vi "OSIPI OPCUA Server.vi"(11 "Main Queue Cluster":T1) -> ()   [LabVIEW 2018]
uses:
  <vilib>/OPCUA/controls/Supported Security Policies.ctl
  Drag and Drop/State Cluster.ctl
  support/Message Queue/Message Cluster.ctl
  Drag and Drop/Thumbnail Cluster.ctl
  Drag and Drop/Object Cluster.ctl
  <vilib>/Utility/miscctls.llb/LVRectTypeDef.ctl
  Drag and Drop/Object Type Enum.ctl
  <vilib>/Utility/miscctls.llb/LVPositionTypeDef.ctl
  Config Module/Controls/Main Config Cluster.ctl
  OPC Module Config.ctl
  Scale Module Folder/Measure Instrument/State Enum.ctl
  <vilib>/Utility/miscctls.llb/LVPoint32TypeDef.ctl
  OPC Settings.ctl
  Variable Data Cluster.ctl
  <vilib>/OPCUA/controls/NodeId.ctl
  <vilib>/OPCUA/controls/OPC UA StatusCode.ctl
  <vilib>/OPCUA/controls/Subscription ID.ctl
  <vilib>/OPCUA/controls/OPC UA Client Refnum.ctl
  <vilib>/OPCUA/controls/Subscription Data Change.ctl
  <vilib>/OPCUA/controls/Data Type.ctl
  Feed Module/Controls/Feed Module Config Cluster.ctl
  Feed Module/Controls/Feed Module Settings Cluster.ctl
  Ismatec ISM 831C/Controls/Ismatech Settings Cluster.ctl
  Masterflex 7550-30/Controls/Settings Cluster.ctl
  Mettler Toledo/Controls/Settings Cluster.ctl
  Bronkhorst M13 Flow Meter/Settings Cluster.ctl
  Measure Instrument/PID 2 Parameters Cluster.ctl
  Measure Instrument/PID Input Enum.ctl
  Measure Instrument/PID 2 Output Enum.ctl
  Tacmina QI/Tacmina QI DAQ Setting.ctl
  KNF Pump/Settings Cluster plus SIMDOS.ctl
  ASIA Pump/Pump Settings.ctl
  VICI M50 Party Mode/Settings Cluster.ctl
  FLOM Pump/Settings Cluster.ctl
  SSI PR Class/SSI PR or LD Settings Cluster.ctl
  Masterflex 75211/Masterflex 75211 DAQ Setting.ctl
  SSI PR Class/SSI P40 Settings Cluster.ctl
  TT Module/Controls/TT Module Config Cluster.ctl
  Tag VIs/Numeric Alarm Settings Cluster.ctl
  Acquisition/Hardware Configuration.ctl
  Acquisition/Task Cluster.ctl
  PT Module/Controls/PT Module Config Cluster.ctl
  Scale Module Folder/Feed Module/Controls/Scale Module Config Cluster.ctl
  Scale Module Folder/Feed Module/Controls/Scale Module Settings Cluster.ctl
  Pump Module Folder/Pump Module Config Cluster.ctl
  Pump Module Folder/Pump Module Settings Cluster.ctl
  LabJack Module/Controls/U3 Module Config Cluster.ctl
  Decoration Module/Decoration Module Config Cluster.ctl
  Flow Module Folder/Feed Module/Controls/Flow Module Config Cluster.ctl
  Flow Module Folder/Feed Module/Controls/Flow Module Settings Cluster.ctl
  TCU Module/TCU Module Folder/TCU Module Config Cluster.ctl
  TCU Module/TCU Module Folder/TCU Module Settings Cluster.ctl
  TCU Module/TCU Module Folder/Measure Instrument/Output Devices.ctl
  Huber TCU/Huber Settings.ctl
  Lauda Integral XT-150 TCU/Lauda Settings.ctl
  Julabo Type 1 TCU/Julabo Type 1 TCU Folder/Julabo FP-50 Settings.ctl
  Huber Unistat 410 TCU/Huber Unistat 410 RS485 Settings.ctl
  D-O Module Folder/Not Sure Where this is Used.ctl
  Sequencing/Squence Control.ctl
  D-O Module Folder/D-O Module Config Cluster.ctl
  D-O Module Folder/Valve Clusters.ctl
  D-O Module Folder/D-O Module Settings Cluster.ctl
  D-O Module Folder/D-O Device Settings Cluster.ctl
  VICI Electronic Actuator/VICI Electronic Actuator Settings.ctl
  Pressure Regulator Control Module/Pressure Regulator/Controls/4-20mA Module Config Cluster.ctl
  Pressure Regulator Control Module/Pressure Regulator/Controls/4-20mA Module Settings Cluster.ctl
  Pressure Transmitter/Pressure Transmitter Device Settings.ctl
  Pressure Reg Module/Pressure Regulator Device Settings.ctl
  <vilib>/OPCUA/controls/OPC UA Variable Node Refnum.ctl
  <vilib>/OPCUA/controls/OPC UA Server Refnum.ctl
  Main/Main Queue Cluster.ctl
  Tag VIs/Tag FGV Operation Enum.ctl
  <vilib>/OPCUA/server/Write Double.vi
  <vilib>/OPCUA/NI OPC UA Server.lvlib
  support/Message Queue/Message Queue.lvlib
  Shared Variables/Dynamic Shared Variables.lvlib
  support/Message Queue/Enqueue Message (Single).vi
  TT Module/TT Module.lvlib
  Masterflex 7550-30/Masterflex 7550-30.lvlib
  Ismatec ISM 831C/Ismatec ISM 831C.lvlib
  Tacmina QI/Tacmina QI.lvlib
  KNF Pump/KNF SIMDOS.lvlib
  VICI M50 Party Mode/VICI M6 M50 Party Mode.lvlib
  FLOM Pump/FLOM Pump.lvlib
  ASIA Pump.lvlib
  Mettler Toledo/Mettler Toledo.lvlib
  Bronkhorst M13 Flow Meter/Bronkhorst M13 Flow Meter.lvlib
  SSI PR Class/SSI PR or LD Pump.lvlib
  Feed Module/Feed Module.lvlib
  DAQ/DAQ.lvlib
  PT Module/PT Module.lvlib
  Scale Module Folder/Scale Module.lvlib
  Pump Module Folder/Pump Module.lvlib
  LabJack Module/U3 Module.lvlib
  Flow Module Folder/Flow Module.lvlib
  Huber TCU/Huber Ministat 230 TCU.lvlib
  Lauda Integral XT-150 TCU/Lauda TCU.lvlib
  Julabo Type 1 TCU/Julabo Type 1 TCU Folder/Julabo Type FP-50 TCU.lvlib
  TCU Module/TCU Module Folder/TCU Module.lvlib
  Sequencing/Sequencing Library.lvlib
  D-O Module Folder/D-O Module.lvlib
  Pressure Transmitter/Pressure Transmitter Library.lvlib
  Pressure Reg Module/Pressure Regulator Library.lvlib
  Pressure Regulator Control Module/Pressure Regulator/4-20mA Module.lvlib
  OPC UA.lvlib
  Scale Module Folder/Measure Instrument/Scale Module Engine.lvlib
  Config Module/Config Module.lvlib
  Drag and Drop/Drag and Drop.lvlib
  D-O Module Folder/DIO Valve/VICI Electronic Actuator.lvlib
  Masterflex 75211/Masterflex 75211.lvlib
  SSI PR Class/SSI P40 Pump.lvlib
  Huber Unistat 410 TCU/Huber Unistat 410 TCU.lvlib
panel:
  out "Array 3":T4(array[cluster])
  out "OPC UA server refnum out 3":T5
  out "Array 2":T6[](array[typedef]) items=["Good"=0, "Good_SubscriptionTransferred"=2949120, "Good_CompletesAsynchronously"=3014656, "Good_Overload"=3080192, "Good_Clamped"=3145728, "Good_LocalOverride"=9830400, "Good_EntryInserted"=10616832, "Good_EntryReplaced"=10682368, "Good_NoData"=10813440, "Good_MoreData"=10878976, "Good_CommunicationEvent"=10944512, "Good_ShutdownEvent"=11010048, "Good_CallAgain"=11075584, "Good_NonCriticalTimeout"=11141120, "Good_ResultsMayBeIncomplete"=12189696, "Good_DataIgnored"=14221312, "Uncertain"=1073741824, "Uncertain_ReferenceOutOfServer"=1080819712, "Uncertain_NoCommunicationLastUsableValue"=1083113472, "Uncertain_LastUsableValue"=1083179008, "Uncertain_SubstituteValue"=1083244544, "Uncertain_InitialValue"=1083310080, "Uncertain_SensorNotAccurate"=1083375616, "Uncertain_EngineeringUnitsExceeded"=1083441152, "Uncertain_SubNormal"=1083506688, "Uncertain_DataSubNormal"=1084489728, "Uncertain_ReferenceNotDeleted"=1086062592, "Uncertain_NotAllNodesAvailable"=1086324736, "Bad"=2147483648, "Bad_UnexpectedError"=2147549184, "Bad_InternalError"=2147614720, "Bad_OutOfMemory"=2147680256, "Bad_ResourceUnavailable"=2147745792, "Bad_CommunicationError"=2147811328, "Bad_EncodingError"=2147876864, "Bad_DecodingError"=2147942400, "Bad_EncodingLimitsExceeded"=2148007936, "Bad_UnknownResponse"=2148073472, "Bad_Timeout"=2148139008, "Bad_ServiceUnsupported"=2148204544, "Bad_Shutdown"=2148270080, "Bad_ServerNotConnected"=2148335616, "Bad_ServerHalted"=2148401152, "Bad_NothingToDo"=2148466688, "Bad_TooManyOperations"=2148532224, "Bad_DataTypeIdUnknown"=2148597760, "Bad_CertificateInvalid"=2148663296, "Bad_SecurityChecksFailed"=2148728832, "Bad_CertificateTimeInvalid"=2148794368, "Bad_CertificateIssuerTimeInvalid"=2148859904, "Bad_CertificateHostNameInvalid"=2148925440, "Bad_CertificateUriInvalid"=2148990976, "Bad_CertificateUseNotAllowed"=2149056512, "Bad_CertificateIssuerUseNotAllowed"=2149122048, "Bad_CertificateUntrusted"=2149187584, "Bad_CertificateRevocationUnknown"=2149253120, "Bad_CertificateIssuerRevocationUnknown"=2149318656, "Bad_CertificateRevoked"=2149384192, "Bad_CertificateIssuerRevoked"=2149449728, "Bad_UserAccessDenied"=2149515264, "Bad_IdentityTokenInvalid"=2149580800, "Bad_IdentityTokenRejected"=2149646336, "Bad_SecureChannelIdInvalid"=2149711872, "Bad_InvalidTimestamp"=2149777408, "Bad_NonceInvalid"=2149842944, "Bad_SessionIdInvalid"=2149908480, "Bad_SessionClosed"=2149974016, "Bad_SessionNotActivated"=2150039552, "Bad_SubscriptionIdInvalid"=2150105088, "Bad_RequestHeaderInvalid"=2150236160, "Bad_TimestampsToReturnInvalid"=2150301696, "Bad_RequestCancelledByClient"=2150367232, "Bad_NoCommunication"=2150694912, "Bad_WaitingForInitialData"=2150760448, "Bad_NodeIdInvalid"=2150825984, "Bad_NodeIdUnknown"=2150891520, "Bad_AttributeIdInvalid"=2150957056, "Bad_IndexRangeInvalid"=2151022592, "Bad_IndexRangeNoData"=2151088128, "Bad_DataEncodingInvalid"=2151153664, "Bad_DataEncodingUnsupported"=2151219200, "Bad_NotReadable"=2151284736, "Bad_NotWritable"=2151350272, "Bad_OutOfRange"=2151415808, "Bad_NotSupported"=2151481344, "Bad_NotFound"=2151546880, "Bad_ObjectDeleted"=2151612416, "Bad_NotImplemented"=2151677952, "Bad_MonitoringModeInvalid"=2151743488, "Bad_MonitoredItemIdInvalid"=2151809024, "Bad_MonitoredItemFilterInvalid"=2151874560, "Bad_MonitoredItemFilterUnsupported"=2151940096, "Bad_FilterNotAllowed"=2152005632, "Bad_StructureMissing"=2152071168, "Bad_EventFilterInvalid"=2152136704, "Bad_ContentFilterInvalid"=2152202240, "Bad_FilterOperandInvalid"=2152267776, "Bad_ContinuationPointInvalid"=2152333312, "Bad_NoContinuationPoints"=2152398848, "Bad_ReferenceTypeIdInvalid"=2152464384, "Bad_BrowseDirectionInvalid"=2152529920, "Bad_NodeNotInView"=2152595456, "Bad_ServerUriInvalid"=2152660992, "Bad_ServerNameMissing"=2152726528, "Bad_DiscoveryUrlMissing"=2152792064, "Bad_SempahoreFileMissing"=2152857600, "Bad_RequestTypeInvalid"=2152923136, "Bad_SecurityModeRejected"=2152988672, "Bad_SecurityPolicyRejected"=2153054208, "Bad_TooManySessions"=2153119744, "Bad_UserSignatureInvalid"=2153185280, "Bad_ApplicationSignatureInvalid"=2153250816, "Bad_NoValidCertificates"=2153316352, "Bad_RequestCancelledByRequest"=2153381888, "Bad_ParentNodeIdInvalid"=2153447424, "Bad_ReferenceNotAllowed"=2153512960, "Bad_NodeIdRejected"=2153578496, "Bad_NodeIdExists"=2153644032, "Bad_NodeClassInvalid"=2153709568, "Bad_BrowseNameInvalid"=2153775104, "Bad_BrowseNameDuplicated"=2153840640, "Bad_NodeAttributesInvalid"=2153906176, "Bad_TypeDefinitionInvalid"=2153971712, "Bad_SourceNodeIdInvalid"=2154037248, "Bad_TargetNodeIdInvalid"=2154102784, "Bad_DuplicateReferenceNotAllowed"=2154168320, "Bad_InvalidSelfReference"=2154233856, "Bad_ReferenceLocalOnly"=2154299392, "Bad_NoDeleteRights"=2154364928, "Bad_ServerIndexInvalid"=2154430464, "Bad_ViewIdUnknown"=2154496000, "Bad_TooManyMatches"=2154627072, "Bad_QueryTooComplex"=2154692608, "Bad_NoMatch"=2154758144, "Bad_MaxAgeInvalid"=2154823680, "Bad_HistoryOperationInvalid"=2154889216, "Bad_HistoryOperationUnsupported"=2154954752, "Bad_WriteNotSupported"=2155020288, "Bad_TypeMismatch"=2155085824, "Bad_MethodInvalid"=2155151360, "Bad_ArgumentsMissing"=2155216896, "Bad_TooManySubscriptions"=2155282432, "Bad_TooManyPublishRequests"=2155347968, "Bad_NoSubscription"=2155413504, "Bad_SequenceNumberUnknown"=2155479040, "Bad_MessageNotAvailable"=2155544576, "Bad_InsufficientClientProfile"=2155610112, "Bad_TcpServerTooBusy"=2155675648, "Bad_TcpMessageTypeInvalid"=2155741184, "Bad_TcpSecureChannelUnknown"=2155806720, "Bad_TcpMessageTooLarge"=2155872256, "Bad_TcpNotEnoughResources"=2155937792, "Bad_TcpInternalError"=2156003328, "Bad_TcpEndpointUrlInvalid"=2156068864, "Bad_RequestInterrupted"=2156134400, "Bad_RequestTimeout"=2156199936, "Bad_SecureChannelClosed"=2156265472, "Bad_SecureChannelTokenUnknown"=2156331008, "Bad_SequenceNumberInvalid"=2156396544, "Bad_ConfigurationError"=2156462080, "Bad_NotConnected"=2156527616, "Bad_DeviceFailure"=2156593152, "Bad_SensorFailure"=2156658688, "Bad_OutOfService"=2156724224, "Bad_DeadbandFilterInvalid"=2156789760, "Bad_RefreshInProgress"=2157379584, "Bad_ConditionAlreadyDisabled"=2157445120, "Bad_ConditionDisabled"=2157510656, "Bad_EventIdUnknown"=2157576192, "Bad_NoData"=2157641728, "Bad_DataLost"=2157772800, "Bad_DataUnavailable"=2157838336, "Bad_EntryExists"=2157903872, "Bad_NoEntryExists"=2157969408, "Bad_TimestampNotSupported"=2158034944, "Bad_InvalidArgument"=2158690304, "Bad_ConnectionRejected"=2158755840, "Bad_Disconnect"=2158821376, "Bad_ConnectionClosed"=2158886912, "Bad_InvalidState"=2158952448, "Bad_EndOfStream"=2159017984, "Bad_NoDataAvailable"=2159083520, "Bad_WaitingForResponse"=2159149056, "Bad_OperationAbandoned"=2159214592, "Bad_ExpectedStreamToBlock"=2159280128, "Bad_WouldBlock"=2159345664, "Bad_SyntaxError"=2159411200, "Bad_MaxConnectionsReached"=2159476736, "Bad_RequestTooLarge"=2159542272, "Bad_ResponseTooLarge"=2159607808, "Bad_EventNotAcknowledgeable"=2159738880, "Bad_InvalidTimestampArgument"=2159869952, "Bad_ProtocolVersionUnsupported"=2159935488, "Bad_StateNotActive"=2160001024, "Bad_FilterOperatorInvalid"=2160132096, "Bad_FilterOperatorUnsupported"=2160197632, "Bad_FilterOperandCountMismatch"=2160263168, "Bad_FilterElementInvalid"=2160328704, "Bad_FilterLiteralInvalid"=2160394240, "Bad_IdentityChangeNotSupported"=2160459776, "Bad_NotTypeDefinition"=2160590848, "Bad_ViewTimestampInvalid"=2160656384, "Bad_ViewParameterMismatch"=2160721920, "Bad_ViewVersionInvalid"=2160787456, "Bad_ConditionAlreadyEnabled"=2160852992, "Bad_DialogNotActive"=2160918528, "Bad_DialogResponseInvalid"=2160984064, "Bad_ConditionBranchAlreadyAcked"=2161049600, "Bad_ConditionBranchAlreadyConfirmed"=2161115136, "Bad_ConditionAlreadyShelved"=2161180672, "Bad_ConditionNotShelved"=2161246208, "Bad_ShelvingTimeOutOfRange"=2161311744, "Bad_AggregateListMismatch"=2161377280, "Bad_AggregateNotSupported"=2161442816, "Bad_AggregateInvalidInputs"=2161508352, "Bad_BoundNotFound"=2161573888, "Bad_BoundNotSupported"=2161639424, "Bad_AggregateConfigurationRejected"=2161770496, "Bad_TooManyMonitoredItems"=2161836032]
  out "OPC UA server refnum out":T5
  out "Array":T4(array[cluster])
  in  "?":T7={"VI refs"=[], "Queues"=[], "[Thumbnails]"=[], "Drag Object Idx"=0, "[Objects]"=[], "Active Object"=0, "Drop Offset"={"Left"=0, "Top"=0}, "Process Name"="", "Main Config"={"Notebook"="", "Page"="", "OPC Module Configs"=[], "Feed Module Configs"=[], "Log File Path"=path "", "TT Module Configs"=[], "DAQ Config"={"Tasks"=[]}, "PT Module Configs"=[], "Scale Module Configs"=[], "Pump Module Configs"=[], "U3 Module Configs"=[{"GUID"="", "Drop Coords"={"Horizontal"=0, "Vertical"=0}, "AI Channel Number"=enum."Default", "Process Name"="", "Queue Name"="", "Input Channel Numeric Alarm Settings"=[]}], "Decoration Module Configs"=[], "Flow Module Configs"=[], "TCU Module Configs"=[], "Steps"=[], "Abort"=FALSE, "DO Module Configs"=[], "PR Module Configs"=[], "Cycle Period"=0.0}, "Campaign Filepath"=path "", "Config Changed?"=FALSE} {"Main Config"."PR Module Configs"."Settings"."PID 2 Parameters"."output range"."output low" format="%.2f"; "Main Config"."PR Module Configs"."Settings"."PID 2 Parameters"."output range"."output high" min=0.0 max=100.0 format="%.2f"; "Main Config"."PR Module Configs"."Settings"."PID 2 Parameters"."PID gains"."derivative time (Td, min)" format="%.3f"; "Main Config"."PR Module Configs"."Settings"."PID 2 Parameters"."PID gains"."integral time (Ti, min)" format="%.3f"; "Main Config"."PR Module Configs"."Settings"."PID 2 Parameters"."PID gains"."proportional gain (Kc)" format="%.3f"; "Main Config"."Steps"."Control" items=["Pump %", "Setpoint"]; "Main Config"."TCU Module Configs"."Settings"."Huber Unistat 410 Settings"."Address" min=0 max=99 format="%02.0f"; "Main Config"."TCU Module Configs"."Settings"."Julabo FP-50 Settings"."Pump Power" min=0 max=8 step=1; "Main Config"."TCU Module Configs"."Settings"."Lauda Settings"."Pump Power" min=0 max=8 step=1; "Main Config"."Pump Module Configs"."Settings"."ASIA Pump C"."channel" min=0 max=1 step=1; "Main Config"."Pump Module Configs"."Settings"."Masterflex"."Pump Number" min=1.0 max=20.0 step=1.0; "Main Config"."Pump Module Configs"."Settings"."Ismatech"."Pump Number" min=1.0 max=20.0 step=1.0; "Main Config"."Feed Module Configs"."Settings"."output range"."output low" min=0.0 max=100.0 format="%.2f"; "Main Config"."Feed Module Configs"."Settings"."output range"."output high" format="%.2f"; "Main Config"."Feed Module Configs"."Settings"."PID 2 Parameters"."PID gains"."derivative time (Td, min)" format="%.3f"; "Main Config"."Feed Module Configs"."Settings"."PID 2 Parameters"."PID gains"."integral time (Ti, min)" format="%.3f"; "Main Config"."Feed Module Configs"."Settings"."PID 2 Parameters"."PID gains"."proportional gain (Kc)" format="%.3f"; "Main Config"."Feed Module Configs"."Settings"."ASIA Pump C"."channel" min=0 max=1 step=1; "Main Config"."Feed Module Configs"."Settings"."Ismatech"."Pump Number" min=1.0 max=20.0 step=1.0; "Main Config"."Feed Module Configs"."Settings"."Masterflex"."Pump Number" min=1.0 max=20.0 step=1.0}
  out "Tag Values":dbl[](array[numeric])
  out "Tag Names":string[](array[string])
  in  "?":T7 {"Main Config"."PR Module Configs"."Settings"."PID 2 Parameters"."output range"."output low" format="%.2f"; "Main Config"."PR Module Configs"."Settings"."PID 2 Parameters"."output range"."output high" min=0.0 max=100.0 format="%.2f"; "Main Config"."PR Module Configs"."Settings"."PID 2 Parameters"."PID gains"."derivative time (Td, min)" format="%.3f"; "Main Config"."PR Module Configs"."Settings"."PID 2 Parameters"."PID gains"."integral time (Ti, min)" format="%.3f"; "Main Config"."PR Module Configs"."Settings"."PID 2 Parameters"."PID gains"."proportional gain (Kc)" format="%.3f"; "Main Config"."Steps"."Control" items=["Pump %", "Setpoint"]; "Main Config"."TCU Module Configs"."Settings"."Huber Unistat 410 Settings"."Address" min=0 max=99 format="%02.0f"; "Main Config"."TCU Module Configs"."Settings"."Julabo FP-50 Settings"."Pump Power" min=0 max=8 step=1; "Main Config"."TCU Module Configs"."Settings"."Lauda Settings"."Pump Power" min=0 max=8 step=1; "Main Config"."Pump Module Configs"."Settings"."ASIA Pump C"."channel" min=0 max=1 step=1; "Main Config"."Pump Module Configs"."Settings"."Masterflex"."Pump Number" min=1.0 max=20.0 step=1.0; "Main Config"."Pump Module Configs"."Settings"."Ismatech"."Pump Number" min=1.0 max=20.0 step=1.0; "Main Config"."Feed Module Configs"."Settings"."output range"."output low" min=0.0 max=100.0 format="%.2f"; "Main Config"."Feed Module Configs"."Settings"."output range"."output high" format="%.2f"; "Main Config"."Feed Module Configs"."Settings"."PID 2 Parameters"."PID gains"."derivative time (Td, min)" format="%.3f"; "Main Config"."Feed Module Configs"."Settings"."PID 2 Parameters"."PID gains"."integral time (Ti, min)" format="%.3f"; "Main Config"."Feed Module Configs"."Settings"."PID 2 Parameters"."PID gains"."proportional gain (Kc)" format="%.3f"; "Main Config"."Feed Module Configs"."Settings"."ASIA Pump C"."channel" min=0 max=1 step=1; "Main Config"."Feed Module Configs"."Settings"."Ismatech"."Pump Number" min=1.0 max=20.0 step=1.0; "Main Config"."Feed Module Configs"."Settings"."Masterflex"."Pump Number" min=1.0 max=20.0 step=1.0}
  in  "supported security policies (None)":T69={"None"=TRUE, "Sign with Basic128Rsa15"=TRUE, "Sign and Encrypt with Basic128Rsa15"=TRUE, "Sign with Basic256"=TRUE, "Sign and Encrypt with Basic256"=TRUE}
  out "server endpoint URL":string
  # "Instrument Settings"
  # "Instrument Settings"
  # "Output Instruments"
  # "Flow Meter Settings"
  # "Output Instruments"
  # "Scale Settings"
  # "Output Instruments"
  # "Input Instruments"
  # "Instrument Settings"
  # "Instrument Settings"
  # "Output Instruments"
  # "Flow Meter Settings"
  # "Output Instruments"
  # "Scale Settings"
  # "Output Instruments"
  # "Input Instruments"
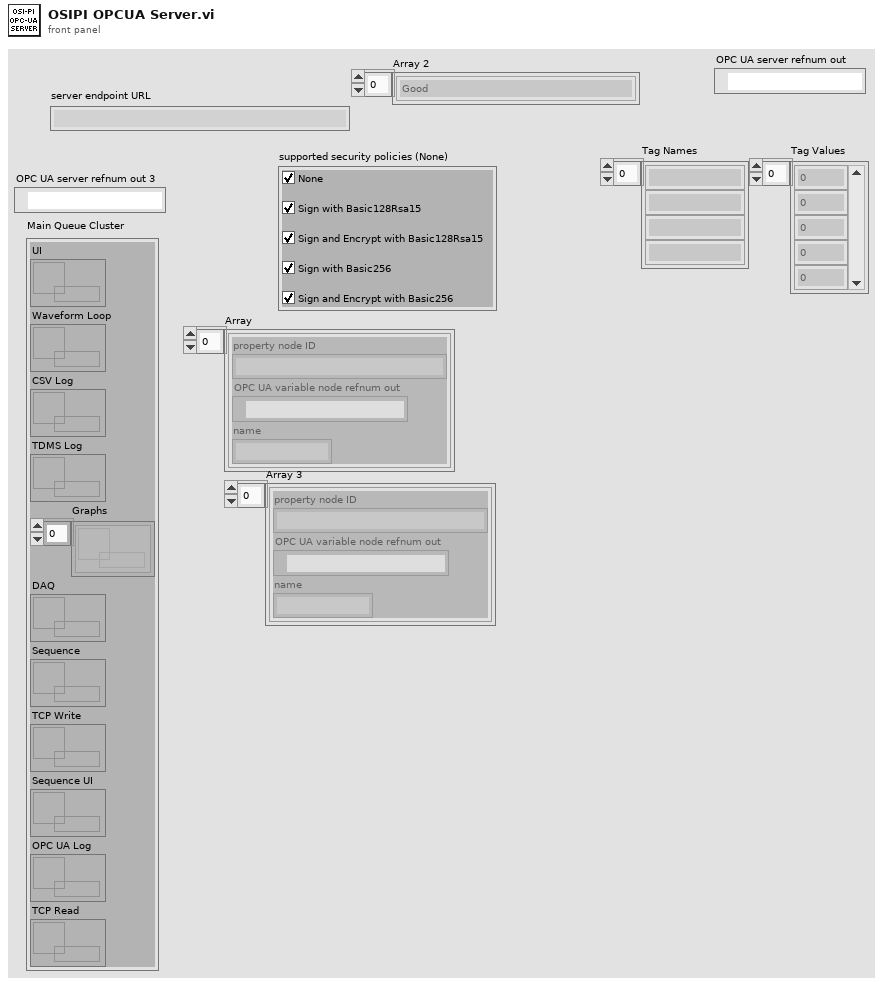
[diagram p1: front panel]
types:
  T1 = typedef "Main Queue Cluster.ctl" = cluster{"UI":refnum<queue>, "Waveform Loop":refnum<queue>, "CSV Log":refnum<queue>, "TDMS Log":refnum<queue>, "Graphs":refnum<queue>[], "DAQ":refnum<queue>, "Sequence":refnum<queue>, "TCP Write":refnum<queue>, "Sequence UI":refnum<queue>, "OPC UA Log":refnum<queue>, "TCP Read":refnum<queue>}
  T2 = typedef "NodeId.ctl" = string
  T3 = typedef "OPC UA Variable Node Refnum.ctl" = refnum<k21>
  T4 = cluster{"property node ID":T2, "OPC UA variable node refnum out":T3, "name":string}[]
  T5 = typedef "OPC UA Server Refnum.ctl" = refnum<k21>
  T6 = typedef "OPC UA StatusCode.ctl" = u32
  T7 = typedef "Drag and Drop.lvlib/State Cluster.ctl" = cluster{"VI refs":refnum<vi>[], "Queues":refnum<queue>[], "[Thumbnails]":T8[], "Drag Object Idx":i32, "[Objects]":T9[], "Active Object":i32, "Drop Offset":T12, "Process Name":string, "Main Config":T13, "Campaign Filepath":path, "Config Changed?":bool}
  T8 = typedef "Thumbnail Cluster.ctl" = cluster{"Path":path, "Rectangle":cluster{"left":i16, "top":i16, "right":i16, "bottom":i16}}
  T9 = typedef "Object Cluster.ctl" = cluster{"BMP Path":path, "Anchor Position":cluster{"X":i32, "Y":i32}, "Hot Spot":T10, "Type":T11, "Parameters":variant}
  T10 = typedef "LVRectTypeDef.ctl" = cluster{"Left":i16, "Top":i16, "Right":i16, "Bottom":i16}
  T11 = typedef "Object Type Enum.ctl" = enum16{"Icon", "Line", "Text", "Feed Module"}
  T12 = typedef "LVPositionTypeDef.ctl" = cluster{"Left":i32, "Top":i32}
  T13 = typedef "Config Module.lvlib/Main Config Cluster.ctl" = cluster{"Notebook":string, "Page":string, "OPC Module Configs":T14[], "Feed Module Configs":T21[], "Log File Path":path, "TT Module Configs":T38[], "DAQ Config":T40, "PT Module Configs":T42[], "Scale Module Configs":T43[], "Pump Module Configs":T45[], "U3 Module Configs":T47[], "Decoration Module Configs":T48[], "Flow Module Configs":T49[], "TCU Module Configs":T51[], "Steps":T58, "Abort":bool, "DO Module Configs":T60[], "PR Module Configs":T65[], "Cycle Period":dbl}
  T14 = typedef "OPC UA.lvlib/OPC Module Config.ctl" = cluster{"State":T15, "GUID":string, "Drop Coords":T16, "Configuration":T17, "First Iteration":bool, "Data":cluster{"Object Name":string, "Variable Array":T18[]}[], "Process Name":string, "Load Count":i32, "Log Started":bool, "subscription ID out":T19, "OPC UA client refnum out":T20, "Event Registration Refnum":refnum<event-registration>, "Start Time":timestamp, "Current Time":timestamp}
  T15 = typedef "Scale Module.lvlib/Scale Module Engine.lvlib/State Enum.ctl" = enum16{"Measuring", "Idle"}
  T16 = typedef "LVPoint32TypeDef.ctl" = cluster{"Horizontal":i32, "Vertical":i32}
  T17 = typedef "OPC UA.lvlib/OPC Settings.ctl" = cluster{"Cycle Period":dbl, "server endpoint URL":string, "security policy":cluster{"message mode":enum16{"None", "Sign", "Sign and Encrypt"}, "security":enum16{"Basic256", "Basic128Rsa15"}}, "Trust Any Server":bool}
  T18 = typedef "OPC UA.lvlib/Variable Data Cluster.ctl" = cluster{"node ID":T2, "browse name":string, "status":T6, "timestamp":timestamp, "value ":variant}
  T19 = typedef "Subscription ID.ctl" = u32
  T20 = typedef "OPC UA Client Refnum.ctl" = refnum<k21>
  T21 = typedef "Feed Module.lvlib/Feed Module Config Cluster.ctl" = cluster{"GUID":string, "Drop Coords":T16, "Process Name":string, "Queue Name":string, "Settings":T22, "Settings Load Count":i32, "OP Load Count":i32}
  T22 = typedef "Feed Module.lvlib/Feed Module Settings Cluster.ctl" = cluster{"Cycle Period":dbl, "Ismatech":T23, "Masterflex":T24, "Mettler":T25, "Bronkhorst M13 Flow Meter":T26, "PID 2 Parameters":T27, "Manual Entry":dbl, "Auto?":bool, "output range":cluster{"output high":dbl, "output low":dbl}, "Bronkhorst M14":T25, "Tacmina Settings":T30, "KNF SIMDOS Settings":T31, "ASIA Pump C":T32, "VICI Settings":T33, "FLOM Settings":T34, "SSI PR/LD Settings":T35, "Masterflex 75211 Settings":T36, "SSI P40 Settings":T37}
  T23 = typedef "Ismatec ISM 831C.lvlib/Ismatech Settings Cluster.ctl" = cluster{"VISA resource name":refnum<visa-resource-name>, "Simulated?":bool, "Pump Number":dbl, "Reverse?":bool}
  T24 = typedef "Masterflex 7550-30.lvlib/Settings Cluster.ctl" = cluster{"VISA resource name":refnum<visa-resource-name>, "Simulated?":bool, "Pump Number":dbl, "Reverse?":bool}
  T25 = typedef "Mettler Toledo.lvlib/Settings Cluster.ctl" = cluster{"VISA resource name":refnum<visa-resource-name>, "Simulated?":bool}
  T26 = typedef "Bronkhorst M13 Flow Meter.lvlib/Settings Cluster.ctl" = cluster{"VISA resource name":refnum<visa-resource-name>, "Simulated?":bool}
  T27 = typedef "PID 2 Parameters Cluster.ctl" = cluster{"Input Device":T28, "Output Device":T29, "Setpoint":dbl, "PID gains":cluster{"proportional gain (Kc)":dbl, "integral time (Ti, min)":dbl, "derivative time (Td, min)":dbl}}
  T28 = typedef "PID Input Enum.ctl" = enum16{"Default", "Bronkhorst M13", "Bronkhorst M14", "Scale Rate of Change"}
  T29 = typedef "PID 2 Output Enum.ctl" = enum16{"Default", "Ismatec ISM 831C", "Masterflex 7550-30", "VICI", "Tacmina QI", "KNF SIMDOS", "ASIA Type C", "FLOM UI-22-11", "SSI PR/LD", "SSI P40", "Masterflex 75211-70"}
  T30 = typedef "Tacmina QI.lvlib/Tacmina QI DAQ Setting.ctl" = cluster{"Analog DAQ Task":refnum<k21>, "Digital DAQ Task":refnum<k21>}
  T31 = typedef "KNF SIMDOS.lvlib/Settings Cluster plus SIMDOS.ctl" = cluster{"VISA resource name":refnum<visa-resource-name>, "Simulated?":bool}
  T32 = typedef "ASIA Pump.lvlib/Pump Settings.ctl" = cluster{"ASIA Pump #":i32, "channel":i32, "Simulated":bool}
  T33 = typedef "VICI M6 M50 Party Mode.lvlib/Settings Cluster.ctl" = cluster{"VISA resource name":refnum<visa-resource-name>, "Simulated?":bool, "Pump Letter":string, "Reverse?":bool}
  T34 = typedef "FLOM Pump.lvlib/Settings Cluster.ctl" = cluster{"VISA resource name":refnum<visa-resource-name>, "Simulated?":bool, "Pump Number":dbl}
  T35 = typedef "SSI PR or LD Pump.lvlib/SSI PR or LD Settings Cluster.ctl" = cluster{"VISA resource name":refnum<visa-resource-name>, "Simulated?":bool}
  T36 = typedef "Masterflex 75211.lvlib/Masterflex 75211 DAQ Setting.ctl" = cluster{"Analog DAQ Task":refnum<k21>, "Digital DAQ Task":refnum<k21>}
  T37 = typedef "SSI P40 Pump.lvlib/SSI P40 Settings Cluster.ctl" = cluster{"VISA resource name":refnum<visa-resource-name>, "Simulated?":bool}
  T38 = typedef "TT Module.lvlib/TT Module Config Cluster.ctl" = cluster{"GUID":string, "Drop Coords":T16, "Input Channel Tag Name ":string, "Process Name":string, "Queue Name":string, "Input Channel Numeric Alarm Settings":T39[]}
  T39 = typedef "Numeric Alarm Settings Cluster.ctl" = cluster{"enable? (F)":bool, "name":string, "alarm type":enum16{"HI_HI", "HI", "LO", "LO_LO"}, "level/change":dbl, "deadband/time":dbl, "alarm delay":dbl, "priority":u32, "ack type":enum16{"Auto", "User", "None", "Each Occurrence"}, "area":string, "description":string, "log? (T)":bool}
  T40 = typedef "DAQ.lvlib/Hardware Configuration.ctl" = cluster{"Tasks":T41[]}
  T41 = typedef "Task Cluster.ctl" = cluster{"DAQmx Task":refnum<k21>, "Read-Write Radio":enum32{"Read", "Write"}}
  T42 = typedef "PT Module.lvlib/PT Module Config Cluster.ctl" = cluster{"GUID":string, "Drop Coords":T16, "Input Channel Tag Name ":string, "Process Name":string, "Queue Name":string, "Input Channel Numeric Alarm Settings":T39[]}
  T43 = typedef "Scale Module.lvlib/Scale Module Config Cluster.ctl" = cluster{"GUID":string, "Drop Coords":T16, "Process Name":string, "Queue Name":string, "Settings":T44, "Load Count":i32}
  T44 = typedef "Scale Module.lvlib/Scale Module Settings Cluster.ctl" = cluster{"Cycle Period":dbl, "Mettler":T25, "Scale Type":string}
  T45 = typedef "Pump Module.lvlib/Pump Module Config Cluster.ctl" = cluster{"GUID":string, "Drop Coords":T16, "Process Name":string, "Queue Name":string, "Settings":T46, "Load Count":i32}
  T46 = typedef "Pump Module.lvlib/Pump Module Settings Cluster.ctl" = cluster{"Cycle Period":dbl, "Manual Entry":dbl, "Output Device":T29, "Ismatech":T23, "Masterflex":T24, "VICI Settings":T33, "Tacmina Settings":T30, "KNF SIMDOS Settings":T31, "ASIA Pump C":T32, "FLOM Settings":T34, "SSI PR/LD Settings":T35, "SSI P40 Settings":T35, "Masterflex 75211 Settings":T36, "Pump Calibration File":path, "Calibration Slope":dbl, "Calibration Y Intercept":dbl, "Pump Cal Enum":u16}
  T47 = typedef "U3 Module.lvlib/U3 Module Config Cluster.ctl" = cluster{"GUID":string, "Drop Coords":T16, "AI Channel Number":enum16{"Default", "AI0", "AI1", "AI2", "AI3", "AI4", "AI5", "AI6", "AI7"}, "Process Name":string, "Queue Name":string, "Input Channel Numeric Alarm Settings":T39[]}
  T48 = typedef "Decoration Module Config Cluster.ctl" = cluster{"GUID":string, "Drop Coords":T16, "Decoration Filepath":path}
  T49 = typedef "Flow Module.lvlib/Flow Module Config Cluster.ctl" = cluster{"GUID":string, "Drop Coords":T16, "Process Name":string, "Queue Name":string, "Settings":T50, "Load Count":i32}
  T50 = typedef "Flow Module.lvlib/Flow Module Settings Cluster.ctl" = cluster{"Cycle Period":dbl, "Bronkhorst M13":T25, "Flow Meter Type":string, "Bronkhorst M14":T25}
  T51 = typedef "TCU Module.lvlib/TCU Module Config Cluster.ctl" = cluster{"GUID":string, "Drop Coords":T16, "Process Name":string, "Queue Name":string, "Settings":T52, "Load Count":i32, "Power Level Changed":bool}
  T52 = typedef "TCU Module.lvlib/TCU Module Settings Cluster.ctl" = cluster{"Cycle Period":dbl, "Setpoint Entry":dbl, "Output Device":T53, "Huber Ministat 230 Settings":T54, "Lauda Settings":T55, "Julabo FP-50 Settings":T56, "Internal Control?":bool, "Huber Unistat 410 Settings":T57}
  T53 = typedef "Output Devices.ctl" = enum16{"Default", "Huber Ministat 230", "Huber Unistat 410", "Lauda XT-150", "Julabo FP-50"}
  T54 = typedef "Huber Ministat 230 TCU.lvlib/Huber Settings.ctl" = cluster{"VISA resource name":refnum<visa-resource-name>, "Simulated?":bool}
  T55 = typedef "Lauda TCU.lvlib/Lauda Settings.ctl" = cluster{"VISA resource name":refnum<visa-resource-name>, "Simulated?":bool, "Pump Power":i32}
  T56 = typedef "Julabo Type FP-50 TCU.lvlib/Julabo FP-50 Settings.ctl" = cluster{"VISA resource name":refnum<visa-resource-name>, "Simulated?":bool, "Pump Power":i32}
  T57 = typedef "Huber Unistat 410 TCU.lvlib/Huber Unistat 410 RS485 Settings.ctl" = cluster{"VISA resource name":refnum<visa-resource-name>, "Address":i8, "Simulated?":bool}
  T58 = typedef "Not Sure Where this is Used.ctl" = T59[]
  T59 = typedef "Sequencing Library.lvlib/Squence Control.ctl" = cluster{"Module":string, "Control":u16, "Value":dbl, "Wait (sec)":dbl}
  T60 = typedef "D-O Module.lvlib/D-O Module Config Cluster.ctl" = cluster{"GUID":string, "Drop Coords":T16, "Process Name":string, "Queue Name":string, "Settings":T61, "Load Count":i32}
  T61 = typedef "D-O Module.lvlib/Valve Clusters.ctl" = cluster{"Valve Settings":T62, "Valve Type":enum16{"Default", "Digital Output Valve", "VICI Electronic Actuator"}, "Time On (Sec)":dbl, "Time Off (Sec)":dbl, "Run?":bool}
  T62 = typedef "D-O Module.lvlib/D-O Module Settings Cluster.ctl" = cluster{"D-O Settings":T63, "VICI Electronic Actuator":T64}
  T63 = typedef "D-O Module.lvlib/D-O Device Settings Cluster.ctl" = cluster{"DAQmx Task Name":refnum<k21>, "Output Channel":u16, "Output Channel Names":string[]}
  T64 = typedef "VICI Electronic Actuator.lvlib/VICI Electronic Actuator Settings.ctl" = cluster{"VISA resource name":refnum<visa-resource-name>, "Mode":enum16{"Two Positions With Stops", "Two Positions Without Stops", "Mutiposition"}, "Simulated":bool}
  T65 = typedef "4-20mA Module.lvlib/4-20mA Module Config Cluster.ctl" = cluster{"GUID":string, "Drop Coords":T16, "Process Name":string, "Queue Name":string, "Settings":T66, "Settings Load Count":i32}
  T66 = typedef "4-20mA Module.lvlib/4-20mA Module Settings Cluster.ctl" = cluster{"Cycle Period":dbl, "PID 2 Parameters":cluster{"Input Device":enum16{"Default", "4-20mA"}, "Output Device":enum16{"Default", "Equilibar Pressure Reg", "Flow Regulator"}, "Setpoint":dbl, "PID gains":cluster{"proportional gain (Kc)":dbl, "integral time (Ti, min)":dbl, "derivative time (Td, min)":dbl}, "output range":cluster{"output low":dbl, "output high":dbl}}, "Manual Entry":dbl, "Auto?":bool, "4-20mA Input Settings":T67, "4-20mA Out Settings":T68, "Input Channel Tag Name ":string}
  T67 = typedef "Pressure Transmitter Library.lvlib/Pressure Transmitter Device Settings.ctl" = cluster{"Input Channel ":u16}
  T68 = typedef "Pressure Regulator Library.lvlib/Pressure Regulator Device Settings.ctl" = cluster{"Output DAQ Task":refnum<k21>}
  T69 = typedef "Supported Security Policies.ctl" = cluster{"None":bool, "Sign with Basic128Rsa15":bool, "Sign and Encrypt with Basic128Rsa15":bool, "Sign with Basic256":bool, "Sign and Encrypt with Basic256":bool}
  T70 = typedef "Data Type.ctl" = u16
  T71 = cluster{"name":string, "data type":T70, "access level":u16, "description":string}
  T72 = cluster{"property node ID":T2, "OPC UA variable node refnum out":T3, "name":string}
  T73 = typedef "Tag FGV Operation Enum.ctl" = enum16{"Init", "Set Notification Queue", "Create Tag", "Commit", "Write Tag (Numeric)", "Write Tag (Boolean)", "Read All Tags", "Read One Tag", "Delete Tag Category", "Set Alarm Parameters (Numeric)", "Set Alarm Parameters (Boolean)", "Enable All Alarms", "Disable All Alarms", "Delete All Tags", "Read Alarms", "Ack Alarm", "Read Alarm Parameters (Numeric)", "Read Alarm Parameters (Boolean)"}
  T74 = typedef "Feed Module.lvlib/Feed Module Tag Names Cluster.ctl" = cluster{"Pump Flow Tag":string, "PID 2 Out Tag":string, "Scale Tag":string, "Density Tag":string, "FL Temp":string, "Input Device Tag":string, "Output Device Tag":string, "Pump's Flow":string, "Pump's Pressure":string, "Overpressure Tag":string}
  T75 = typedef "Pump Module.lvlib/Pump Module Tag Names Cluster.ctl" = cluster{"Pump Speed":string, "Pump Flow":string, "Pump Pressure":string, "Output Device Tag":string, "Overpressure Tag":string}
  T76 = typedef "Flow Module.lvlib/Tag Cluster.ctl" = cluster{"Flow Tag":string, "Input Disconnected":string, "Density Tag":string, "Temp Tag":string}
  T77 = typedef "TCU Module.lvlib/TCU Module Tag Names Cluster.ctl" = cluster{"TCU Temp":string, "Output Device Tag":string, "TCU Speed":string}
  T78 = typedef "4-20mA Module.lvlib/4-20mA Module Tag Names Cluster.ctl" = cluster{"4-20mA Input":string, "PID 2 Out Tag":string, "4-20mA Output":string, "Input Device Tag":string, "Output Device Tag":string}
  T79 = cluster{"Feed Module Tags Array":T74[], "DAQ Tags Array":string[], "Scale Tags Array":cluster{"Scale Value":string, "Scale Error":string}[], "Pump Module Tags Array":T75[], "Flow Module Tags Array":T76[], "TCU Module Tags Array":T77[], "PR Module Tags Array":T78[], "OPC Module Tags Array":cluster{"OPC UA Error":string, "Array of Names":string[]}[]}
  T80 = cluster{"Scale Value":string, "Scale Error":string}[]
  T81 = cluster{"OPC UA Error":string, "Array of Names":string[]}[]
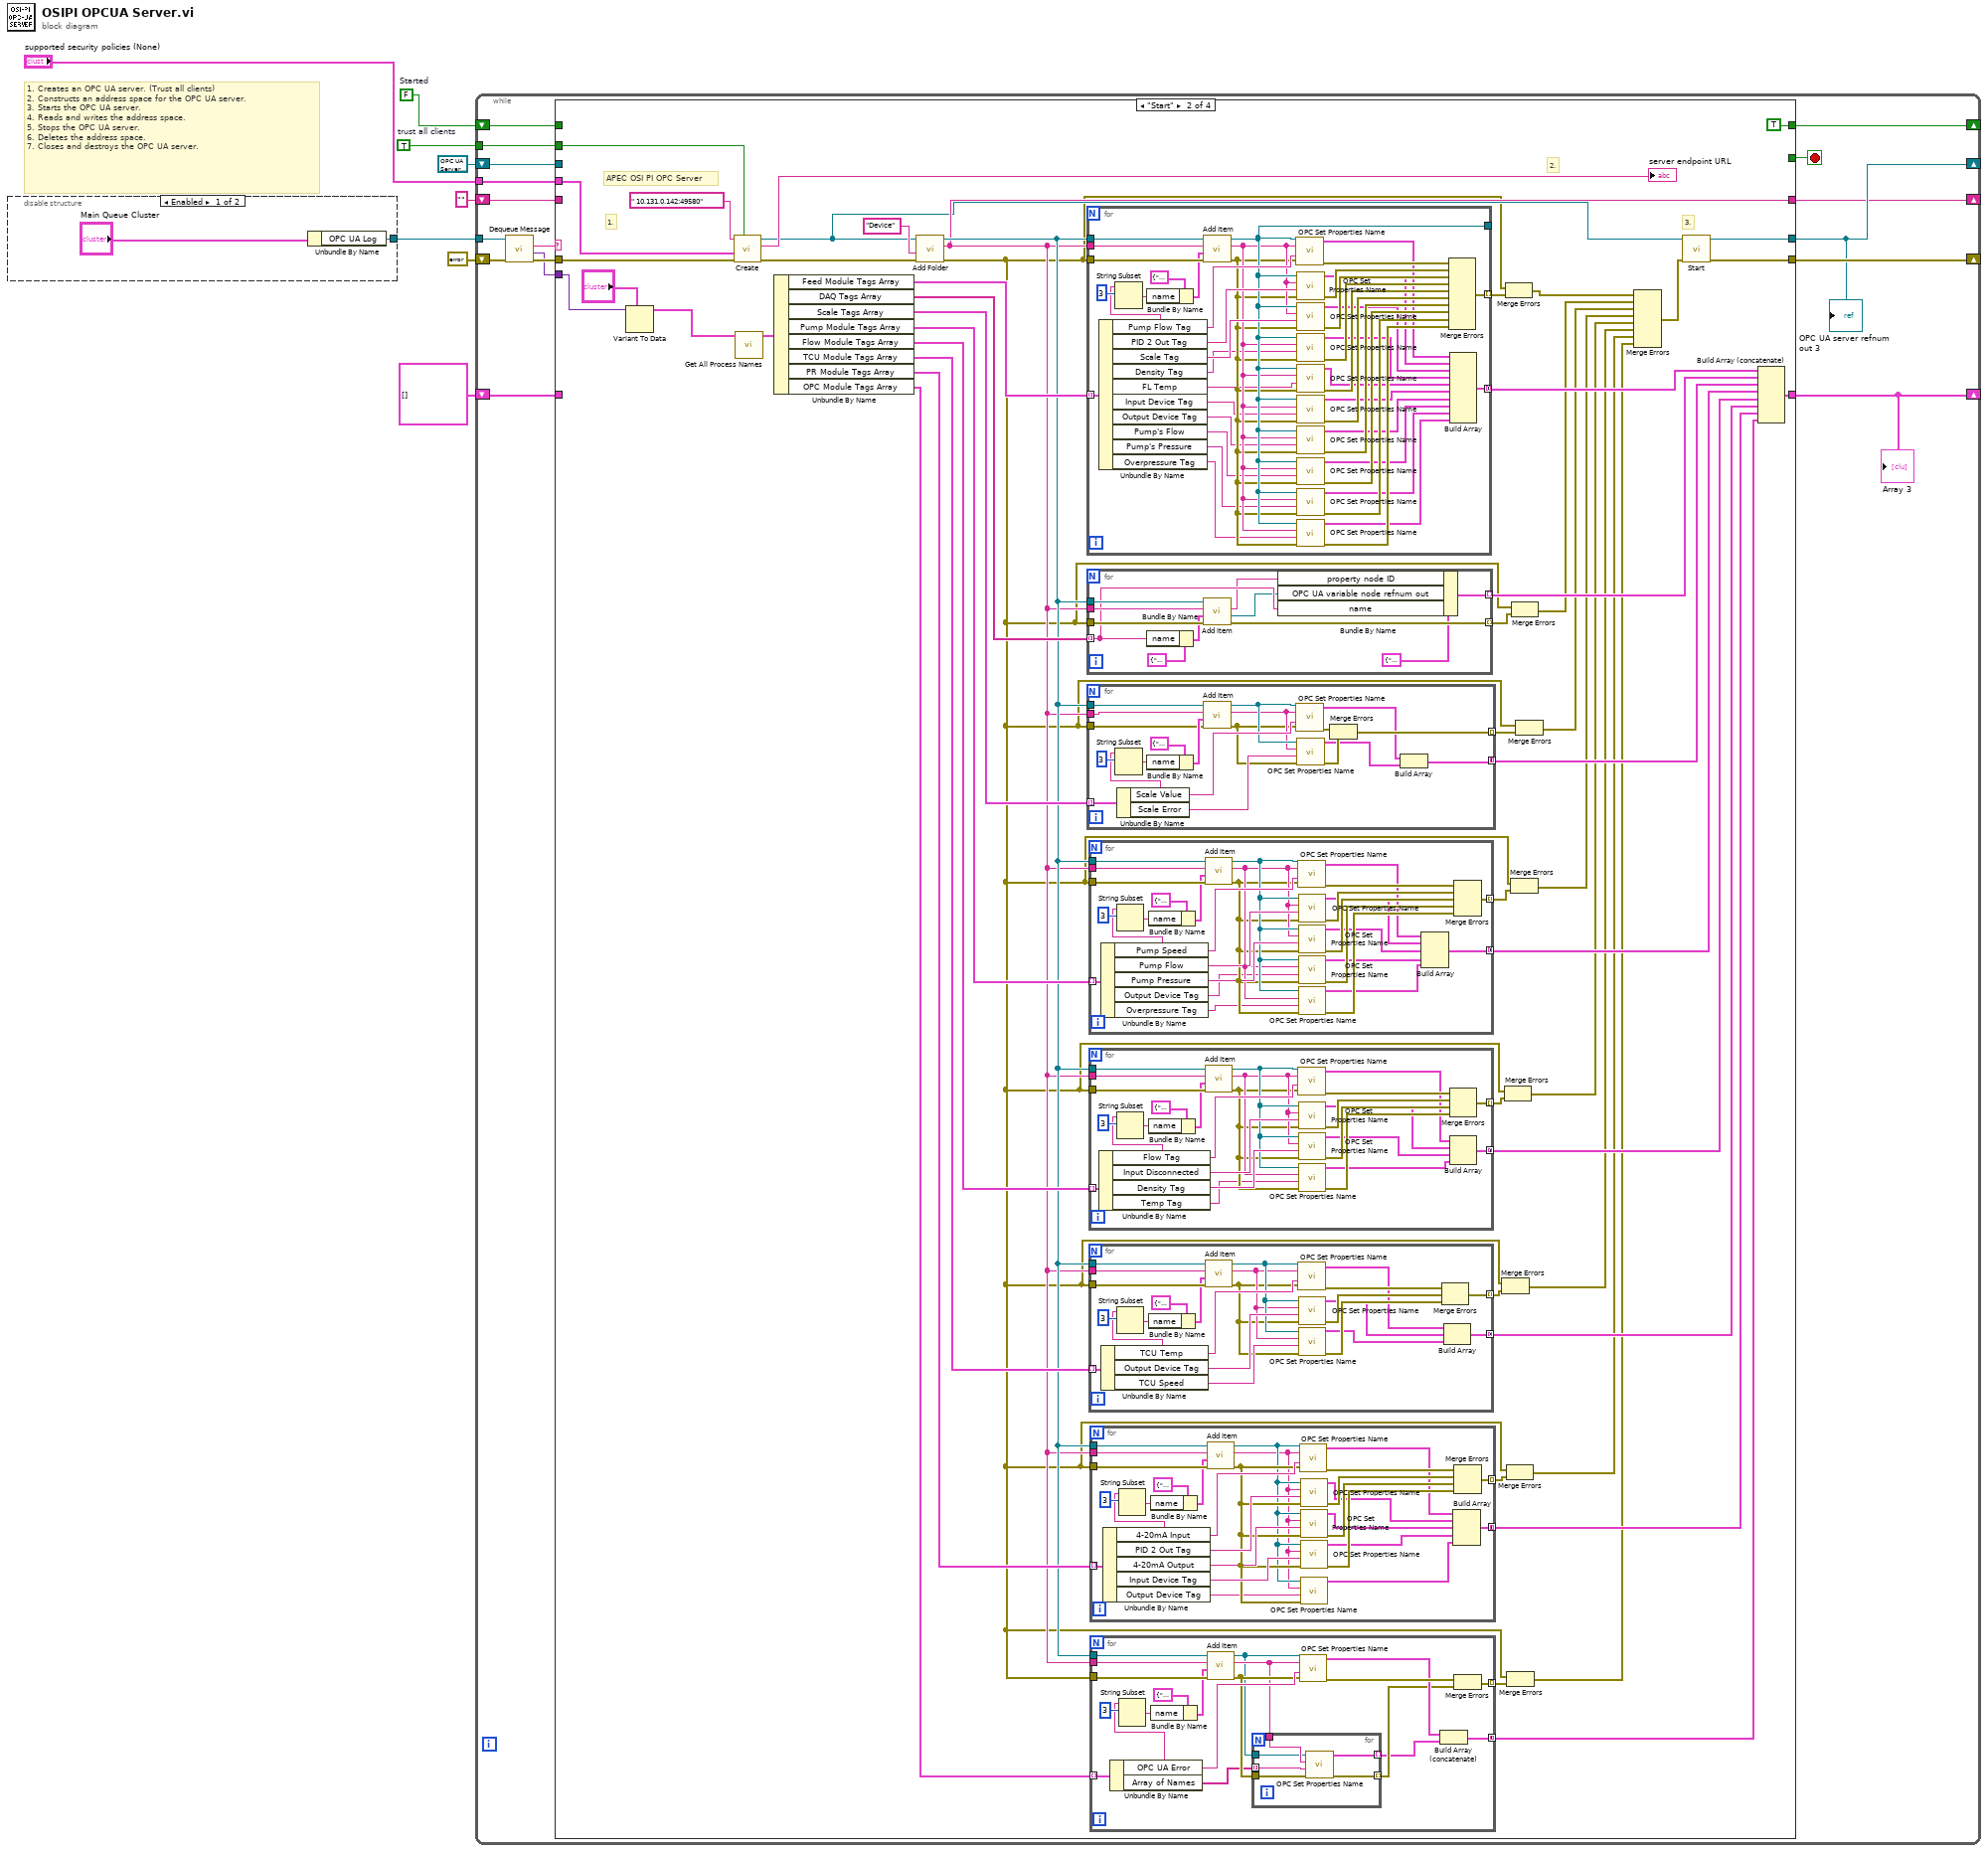
[diagram p0: block diagram]
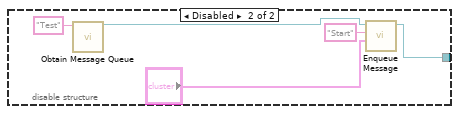
[diagram p2: hidden frame]
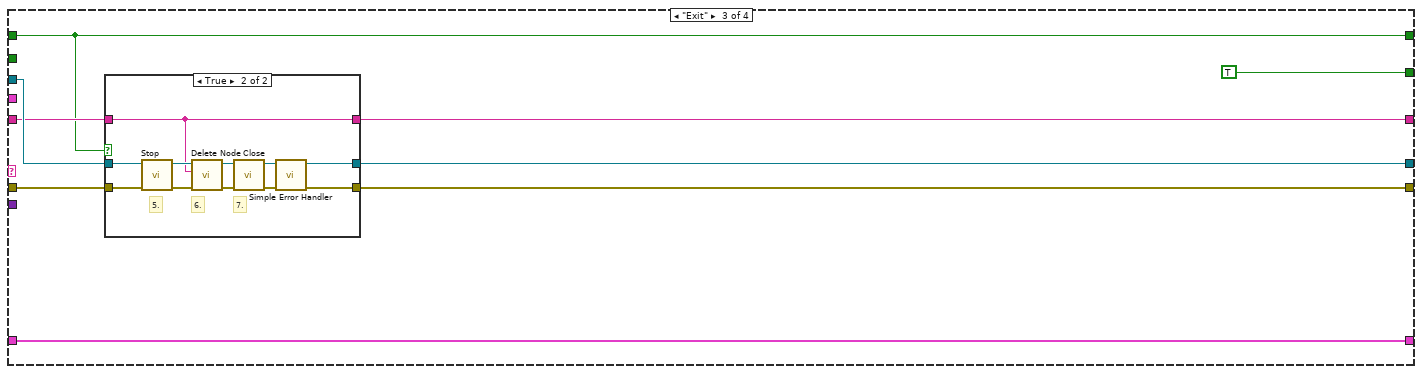
[diagram p4: hidden frame]
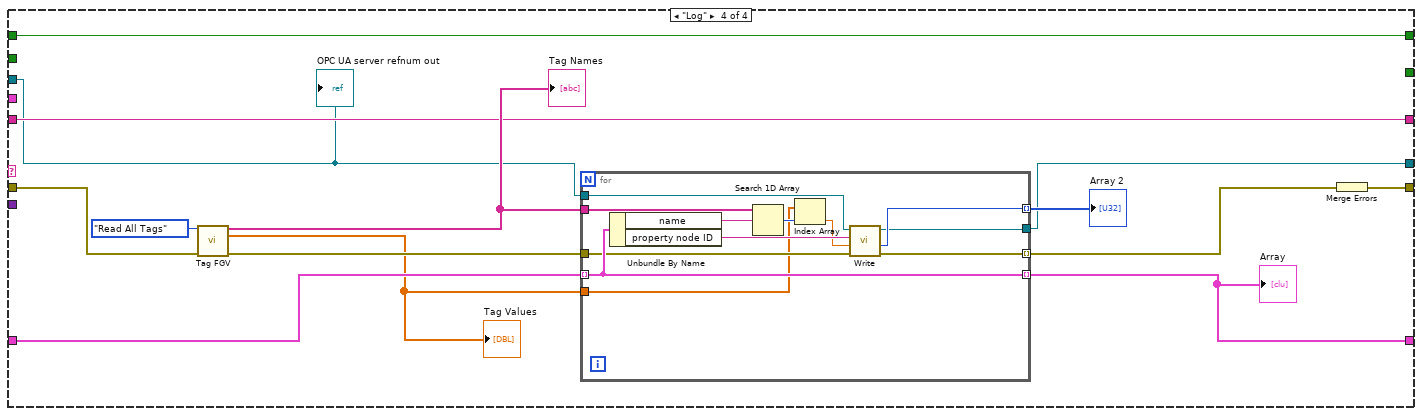
[diagram p6: hidden frame]
diagram:
  w1 = FALSE  # Started
  w8 = TRUE  # trust all clients
  # "1. Creates an OPC UA server. (Trust all clients)\n2. Constructs an address space for the OPC UA server.\n3. Starts the OPC UA server.\n4. Reads and writes the address space.\n5. Stops the OPC UA server.\n6. Deletes the address space.\n7. Closes and destroys the OPC UA server."
  n1 = disable-structure shown="Enabled" {
    disable-tunnel: [w10 w12] -> w6
    frame Enabled {
      n2 = Unbundle By Name("Main Queue Cluster") -> ("OPC UA Log"=w10:refnum<queue>)
    }
    frame Disabled {
      n3 = call "Obtain Message Queue.vi"("name (unnamed)"="Test") -> ("Message Queue"=w11:refnum<queue>)  [unwired: 9 in, 1 out]
      n4 = call-poly "Enqueue Message.vi"("Message Data"="?", "Message"="Start", "Message Queue"=w11) -> ("dup Message Queue"=w12:refnum<queue>)  [unwired: 7 in, 1 out]
    }
  }
  n5 = while {
    tunnel: w6 -> [w31]
    shift-right: [w28] -> _
    shift-left: errorcluster {"status"=FALSE, "code"=0, "source"=""} ("error IO") -> [w27]
    tunnel: w8 -> [w26]
    tunnel: "supported security policies (None)" -> [w25]
    shift-right: [w24] -> _
    shift-left: T5 refnum ("OPC UA server refnum out") -> [w23]
    shift-right: [w22] -> _
    shift-left: T2 "" ("folder node ID") -> [w20]
    shift-right: [w19] -> _
    shift-left: T4 [] -> [w18]
    shift-right: [w17] -> _
    shift-left: w1 -> [w16]
    stop <- w30 stop-if-true
    n6 = call "Dequeue Message.vi"("error in (no error)"=w27, "Message Queue"=w31) -> ("error out"=w29:errorcluster, "Message Data"=w21:variant, "Message"=w32:string)  [unwired: 6 in, 1 out]
    n7 = case shown="\"Start\"" w32 {
      tunnel: [_ _ TRUE _] -> w30
      tunnel: w29 -> [w35 w86 w297 w321]
      tunnel: [w35 w84 w296 w315] -> w28
      tunnel: w26 -> [_ w88 _ _]
      tunnel: w25 -> [_ w87 _ _]
      tunnel: [w36 w85 w294 w312] -> w24
      tunnel: w23 -> [w36 _ w295 w317]
      tunnel: [w37 w59 w290 w322] -> w22
      tunnel: w21 -> [_ w81 _ _]
      tunnel: w20 -> [w37 _ w293 w322]
      tunnel: [w34 w64 w292 w318] -> w19
      tunnel: w18 -> [w34 _ w292 w319]
      tunnel: w16 -> [w33 _ w291 w311]
      tunnel: [w33 TRUE ("Started") w291 w311] -> w17
      frame Default {
      }
      frame "Start" {
        # "APEC OSI PI OPC Server"
        # "3."
        # "2."
        # "1."
        n8 = Variant To Data(type="?", Variant=w81) -> (data=w79:T7)  [unwired: 1 in, 1 out]
        n9 = call <vilib>:"Create.vi"("trust all clients (F)"=w88, "error in (no error)"=w86, "supported security policies (None)"=w87, "OPC UA server name"=" 10.131.0.142:49580") -> ("error out"=w83:errorcluster, "server endpoint URL"=→"server endpoint URL":string, "OPC UA server refnum out"=w57:T5)  [unwired: 5 in]
        n10 = call "Get All Process Names.vi"(11:w79) -> ("Module Tags Array Cluster"=w77:T79)  [unwired: 10 in]
        n11 = Unbundle By Name(w77) -> ("Feed Module Tags Array"=w78:T74[], "DAQ Tags Array"=w76:string[], "Scale Tags Array"=w74:T80, "Pump Module Tags Array"=w73:T75[], "Flow Module Tags Array"=w72:T76[], "TCU Module Tags Array"=w71:T77[], "PR Module Tags Array"=w70:T78[], "OPC Module Tags Array"=w58:T81)
        n12 = call <vilib>:"Add Folder.vi"("error in (no error)"=w83, "folder name"="Device", "OPC UA server refnum in"=w57) -> ("error out"=w39:errorcluster, "folder node ID"=w59:T2, "OPC UA server refnum out"=w60:T5)  [unwired: 5 in]
        n13 = for {
          tunnel: w39 -> [w289]
          tunnel: w59 -> [w288]
          tunnel: w60 -> [w287]
          tunnel: [w281] -> w40 mode=indexing
          tunnel: [w274] -> _
          tunnel: w78 -> [w284] mode=indexing
          tunnel: [w247] -> w69 mode=concatenating
          n14 = Unbundle By Name(w284) -> ("Pump Flow Tag"=w279:string, "PID 2 Out Tag"=w278:string, "Scale Tag"=w280:string, "Density Tag"=w271:string, "FL Temp"=w270:string, "Input Device Tag"=w269:string, "Output Device Tag"=w268:string, "Pump's Flow"=w267:string, "Pump's Pressure"=w266:string, "Overpressure Tag"=w265:string)
          n15 = String Subset(string=w279, length (rest)=3 ("length (rest)")) -> (substring=w282:string)  [unwired: 1 in]
          n16 = Bundle By Name(cluster=T71 {"name"="Node", "data type"=12, "access level"=3, "description"=""} ("item"), "name"=w282) -> (w285:T71)
          n17 = call <vilib>:"Add Item.vi"("error in (no error)"=w289, "item"=w285, "parent folder node ID"=w288, "OPC UA server refnum in"=w287) -> ("error out"=w272:errorcluster, "item node ID"=w273:T2, "OPC UA server refnum out"=w274:T5)  [unwired: 3 in, 1 out]
          n18 = call "OPC Set Properties Name.vi"("error in (no error)"=w272, "name"=w279, "item node ID"=w273, "Refnum in"=w274) -> ("error out"=w277:errorcluster, "OPC Property cluster"=w257:T72)  [unwired: 6 in]
          n19 = call "OPC Set Properties Name.vi"("error in (no error)"=w272, "name"=w278, "item node ID"=w273, "Refnum in"=w274) -> ("error out"=w276:errorcluster, "OPC Property cluster"=w256:T72)  [unwired: 6 in]
          n20 = call "OPC Set Properties Name.vi"("error in (no error)"=w272, "name"=w280, "item node ID"=w273, "Refnum in"=w274) -> ("error out"=w275:errorcluster, "OPC Property cluster"=w255:T72)  [unwired: 6 in]
          n21 = call "OPC Set Properties Name.vi"("error in (no error)"=w272, "name"=w271, "item node ID"=w273, "Refnum in"=w274) -> ("error out"=w264:errorcluster, "OPC Property cluster"=w254:T72)  [unwired: 6 in]
          n22 = call "OPC Set Properties Name.vi"("error in (no error)"=w272, "name"=w270, "item node ID"=w273, "Refnum in"=w274) -> ("error out"=w263:errorcluster, "OPC Property cluster"=w253:T72)  [unwired: 6 in]
          n23 = call "OPC Set Properties Name.vi"("error in (no error)"=w272, "name"=w269, "item node ID"=w273, "Refnum in"=w274) -> ("error out"=w262:errorcluster, "OPC Property cluster"=w252:T72)  [unwired: 6 in]
          n24 = call "OPC Set Properties Name.vi"("error in (no error)"=w272, "name"=w268, "item node ID"=w273, "Refnum in"=w274) -> ("error out"=w261:errorcluster, "OPC Property cluster"=w251:T72)  [unwired: 6 in]
          n25 = call "OPC Set Properties Name.vi"("error in (no error)"=w272, "name"=w267, "item node ID"=w273, "Refnum in"=w274) -> ("error out"=w260:errorcluster, "OPC Property cluster"=w250:T72)  [unwired: 6 in]
          n26 = call "OPC Set Properties Name.vi"("error in (no error)"=w272, "name"=w266, "item node ID"=w273, "Refnum in"=w274) -> ("error out"=w259:errorcluster, "OPC Property cluster"=w249:T72)  [unwired: 6 in]
          n27 = call "OPC Set Properties Name.vi"("error in (no error)"=w272, "name"=w265, "item node ID"=w273, "Refnum in"=w274) -> ("error out"=w258:errorcluster, "OPC Property cluster"=w248:T72)  [unwired: 6 in]
          n28 = Merge Errors(w277, w276, w275, w264, w263, w262, w261, w260, w259, w258) -> (w281:errorcluster)
          n29 = Build Array(w257, w256, w255, w254, w253, w252, w251, w250, w249, w248) -> (w247:T4)
        }
        n30 = for {
          tunnel: w39 -> [w246]
          tunnel: w59 -> [w245]
          tunnel: w60 -> [w244]
          tunnel: [w241] -> w42 mode=indexing
          tunnel: w76 -> [w239] mode=indexing
          tunnel: [w236] -> w68 mode=indexing
          n31 = Bundle By Name(cluster=T71 {"name"="Node", "data type"=11, "access level"=3, "description"=""} ("item"), "name"=w239) -> (w242:T71)
          n32 = call <vilib>:"Add Item.vi"("error in (no error)"=w246, "item"=w242, "parent folder node ID"=w245, "OPC UA server refnum in"=w244) -> ("error out"=w241:errorcluster, "OPC UA variable node refnum out"=w238:T3, "item node ID"=w237:T2)  [unwired: 3 in, 1 out]
          n33 = Bundle By Name(cluster=T72 {"property node ID"="", "OPC UA variable node refnum out"="", "name"=""} ("OPC Property cluster"), "property node ID"=w237, "OPC UA variable node refnum out"=w238, "name"=w239) -> (w236:T72)
        }
        n34 = for {
          tunnel: [w230] -> w44 mode=indexing
          tunnel: w74 -> [w233] mode=indexing
          tunnel: w60 -> [w222]
          tunnel: w59 -> [w221]
          tunnel: w39 -> [w220]
          tunnel: [w217] -> w67 mode=concatenating
          n35 = Unbundle By Name(w233) -> ("Scale Value"=w229:string, "Scale Error"=w228:string)
          n36 = String Subset(string=w229, length (rest)=3 ("length (rest)")) -> (substring=w231:string)  [unwired: 1 in]
          n37 = Bundle By Name(cluster=T71 {"name"="Node", "data type"=12, "access level"=3, "description"=""} ("item"), "name"=w231) -> (w234:T71)
          n38 = call <vilib>:"Add Item.vi"("error in (no error)"=w220, "item"=w234, "parent folder node ID"=w221, "OPC UA server refnum in"=w222) -> ("error out"=w223:errorcluster, "item node ID"=w224:T2, "OPC UA server refnum out"=w225:T5)  [unwired: 3 in, 1 out]
          n39 = call "OPC Set Properties Name.vi"("error in (no error)"=w223, "name"=w229, "item node ID"=w224, "Refnum in"=w225) -> ("error out"=w227:errorcluster, "OPC Property cluster"=w219:T72)  [unwired: 6 in]
          n40 = call "OPC Set Properties Name.vi"("error in (no error)"=w223, "name"=w228, "item node ID"=w224, "Refnum in"=w225) -> ("error out"=w226:errorcluster, "OPC Property cluster"=w218:T72)  [unwired: 6 in]
          n41 = Merge Errors(w227, w226) -> (w230:errorcluster)
          n42 = Build Array(w219, w218) -> (w217:T4)
        }
        n43 = for {
          tunnel: w39 -> [w216]
          tunnel: w59 -> [w215]
          tunnel: w60 -> [w214]
          tunnel: [w208] -> w46 mode=indexing
          tunnel: w73 -> [w211] mode=indexing
          tunnel: [w189] -> w66 mode=concatenating
          n44 = Unbundle By Name(w211) -> ("Pump Speed"=w206:string, "Pump Flow"=w205:string, "Pump Pressure"=w207:string, "Output Device Tag"=w198:string, "Overpressure Tag"=w197:string)
          n45 = String Subset(string=w206, length (rest)=3 ("length (rest)")) -> (substring=w209:string)  [unwired: 1 in]
          n46 = Bundle By Name(cluster=T71 {"name"="Node", "data type"=12, "access level"=3, "description"=""} ("item"), "name"=w209) -> (w212:T71)
          n47 = call <vilib>:"Add Item.vi"("error in (no error)"=w216, "item"=w212, "parent folder node ID"=w215, "OPC UA server refnum in"=w214) -> ("error out"=w199:errorcluster, "item node ID"=w200:T2, "OPC UA server refnum out"=w201:T5)  [unwired: 3 in, 1 out]
          n48 = call "OPC Set Properties Name.vi"("error in (no error)"=w199, "name"=w206, "item node ID"=w200, "Refnum in"=w201) -> ("error out"=w204:errorcluster, "OPC Property cluster"=w194:T72)  [unwired: 6 in]
          n49 = call "OPC Set Properties Name.vi"("error in (no error)"=w199, "name"=w205, "item node ID"=w200, "Refnum in"=w201) -> ("error out"=w203:errorcluster, "OPC Property cluster"=w193:T72)  [unwired: 6 in]
          n50 = call "OPC Set Properties Name.vi"("error in (no error)"=w199, "name"=w207, "item node ID"=w200, "Refnum in"=w201) -> ("error out"=w202:errorcluster, "OPC Property cluster"=w192:T72)  [unwired: 6 in]
          n51 = call "OPC Set Properties Name.vi"("error in (no error)"=w199, "name"=w198, "item node ID"=w200, "Refnum in"=w201) -> ("error out"=w196:errorcluster, "OPC Property cluster"=w191:T72)  [unwired: 6 in]
          n52 = call "OPC Set Properties Name.vi"("error in (no error)"=w199, "name"=w197, "item node ID"=w200, "Refnum in"=w201) -> ("error out"=w195:errorcluster, "OPC Property cluster"=w190:T72)  [unwired: 6 in]
          n53 = Build Array(w194, w193, w192, w191, w190) -> (w189:T4)
          n54 = Merge Errors(w204, w203, w202, w196, w195) -> (w208:errorcluster)
        }
        n55 = for {
          tunnel: w39 -> [w188]
          tunnel: w59 -> [w187]
          tunnel: w60 -> [w186]
          tunnel: [w180] -> w48 mode=indexing
          tunnel: w72 -> [w183] mode=indexing
          tunnel: [w164] -> w65 mode=concatenating
          n56 = Unbundle By Name(w183) -> ("Flow Tag"=w178:string, "Input Disconnected"=w177:string, "Density Tag"=w179:string, "Temp Tag"=w170:string)
          n57 = String Subset(string=w178, length (rest)=3 ("length (rest)")) -> (substring=w181:string)  [unwired: 1 in]
          n58 = Bundle By Name(cluster=T71 {"name"="Node", "data type"=12, "access level"=3, "description"=""} ("item"), "name"=w181) -> (w184:T71)
          n59 = call <vilib>:"Add Item.vi"("error in (no error)"=w188, "item"=w184, "parent folder node ID"=w187, "OPC UA server refnum in"=w186) -> ("error out"=w171:errorcluster, "item node ID"=w172:T2, "OPC UA server refnum out"=w173:T5)  [unwired: 3 in, 1 out]
          n60 = call "OPC Set Properties Name.vi"("error in (no error)"=w171, "name"=w178, "item node ID"=w172, "Refnum in"=w173) -> ("error out"=w176:errorcluster, "OPC Property cluster"=w168:T72)  [unwired: 6 in]
          n61 = call "OPC Set Properties Name.vi"("error in (no error)"=w171, "name"=w177, "item node ID"=w172, "Refnum in"=w173) -> ("error out"=w175:errorcluster, "OPC Property cluster"=w167:T72)  [unwired: 6 in]
          n62 = call "OPC Set Properties Name.vi"("error in (no error)"=w171, "name"=w179, "item node ID"=w172, "Refnum in"=w173) -> ("error out"=w174:errorcluster, "OPC Property cluster"=w166:T72)  [unwired: 6 in]
          n63 = call "OPC Set Properties Name.vi"("error in (no error)"=w171, "name"=w170, "item node ID"=w172, "Refnum in"=w173) -> ("error out"=w169:errorcluster, "OPC Property cluster"=w165:T72)  [unwired: 6 in]
          n64 = Merge Errors(w176, w175, w174, w169) -> (w180:errorcluster)
          n65 = Build Array(w168, w167, w166, w165) -> (w164:T4)
        }
        n66 = for {
          tunnel: w39 -> [w163]
          tunnel: w59 -> [w162]
          tunnel: w60 -> [w161]
          tunnel: [w155] -> w50 mode=indexing
          tunnel: w71 -> [w158] mode=indexing
          tunnel: [w142] -> w63 mode=concatenating
          n67 = Unbundle By Name(w158) -> ("TCU Temp"=w153:string, "Output Device Tag"=w152:string, "TCU Speed"=w154:string)
          n68 = String Subset(string=w153, length (rest)=3 ("length (rest)")) -> (substring=w156:string)  [unwired: 1 in]
          n69 = Bundle By Name(cluster=T71 {"name"="Node", "data type"=12, "access level"=3, "description"=""} ("item"), "name"=w156) -> (w159:T71)
          n70 = call <vilib>:"Add Item.vi"("error in (no error)"=w163, "item"=w159, "parent folder node ID"=w162, "OPC UA server refnum in"=w161) -> ("error out"=w146:errorcluster, "item node ID"=w147:T2, "OPC UA server refnum out"=w148:T5)  [unwired: 3 in, 1 out]
          n71 = call "OPC Set Properties Name.vi"("error in (no error)"=w146, "name"=w153, "item node ID"=w147, "Refnum in"=w148) -> ("error out"=w151:errorcluster, "OPC Property cluster"=w145:T72)  [unwired: 6 in]
          n72 = call "OPC Set Properties Name.vi"("error in (no error)"=w146, "name"=w152, "item node ID"=w147, "Refnum in"=w148) -> ("error out"=w150:errorcluster, "OPC Property cluster"=w144:T72)  [unwired: 6 in]
          n73 = call "OPC Set Properties Name.vi"("error in (no error)"=w146, "name"=w154, "item node ID"=w147, "Refnum in"=w148) -> ("error out"=w149:errorcluster, "OPC Property cluster"=w143:T72)  [unwired: 6 in]
          n74 = Merge Errors(w151, w150, w149) -> (w155:errorcluster)
          n75 = Build Array(w145, w144, w143) -> (w142:T4)
        }
        n76 = for {
          tunnel: w39 -> [w141]
          tunnel: w59 -> [w140]
          tunnel: w60 -> [w139]
          tunnel: [w133] -> w52 mode=indexing
          tunnel: w70 -> [w136] mode=indexing
          tunnel: [w115] -> w62 mode=concatenating
          n77 = Unbundle By Name(w136) -> ("4-20mA Input"=w131:string, "PID 2 Out Tag"=w130:string, "4-20mA Output"=w132:string, "Input Device Tag"=w125:string, "Output Device Tag"=w121:string)
          n78 = String Subset(string=w131, length (rest)=3 ("length (rest)")) -> (substring=w134:string)  [unwired: 1 in]
          n79 = Bundle By Name(cluster=T71 {"name"="Node", "data type"=12, "access level"=3, "description"=""} ("item"), "name"=w134) -> (w137:T71)
          n80 = call <vilib>:"Add Item.vi"("error in (no error)"=w141, "item"=w137, "parent folder node ID"=w140, "OPC UA server refnum in"=w139) -> ("error out"=w124:errorcluster, "item node ID"=w122:T2, "OPC UA server refnum out"=w123:T5)  [unwired: 3 in, 1 out]
          n81 = call "OPC Set Properties Name.vi"("error in (no error)"=w124, "name"=w131, "item node ID"=w122, "Refnum in"=w123) -> ("error out"=w129:errorcluster, "OPC Property cluster"=w120:T72)  [unwired: 6 in]
          n82 = call "OPC Set Properties Name.vi"("error in (no error)"=w124, "name"=w130, "item node ID"=w122, "Refnum in"=w123) -> ("error out"=w128:errorcluster, "OPC Property cluster"=w119:T72)  [unwired: 6 in]
          n83 = call "OPC Set Properties Name.vi"("error in (no error)"=w124, "name"=w132, "item node ID"=w122, "Refnum in"=w123) -> ("error out"=w127:errorcluster, "OPC Property cluster"=w118:T72)  [unwired: 6 in]
          n84 = call "OPC Set Properties Name.vi"("error in (no error)"=w124, "name"=w125, "item node ID"=w122, "Refnum in"=w123) -> ("error out"=w126:errorcluster, "OPC Property cluster"=w117:T72)  [unwired: 6 in]
          n85 = call "OPC Set Properties Name.vi"("error in (no error)"=w124, "name"=w121, "item node ID"=w122, "Refnum in"=w123) -> ("OPC Property cluster"=w116:T72)  [unwired: 6 in, 1 out]
          n86 = Build Array(w120, w119, w118, w117, w116) -> (w115:T4)
          n87 = Merge Errors(w129, w128, w127, w126) -> (w133:errorcluster)
        }
        n88 = for {
          tunnel: w39 -> [w108]
          tunnel: w59 -> [w107]
          tunnel: w60 -> [w106]
          tunnel: [w100] -> w54 mode=indexing
          tunnel: w58 -> [w103] mode=indexing
          tunnel: [w96] -> w61 mode=concatenating
          n89 = Unbundle By Name(w103) -> ("OPC UA Error"=w99:string, "Array of Names"=w91:string[])
          n90 = String Subset(string=w99, length (rest)=3 ("length (rest)")) -> (substring=w101:string)  [unwired: 1 in]
          n91 = Bundle By Name(cluster=T71 {"name"="Node", "data type"=12, "access level"=3, "description"=""} ("item"), "name"=w101) -> (w104:T71)
          n92 = call <vilib>:"Add Item.vi"("error in (no error)"=w108, "item"=w104, "parent folder node ID"=w107, "OPC UA server refnum in"=w106) -> ("error out"=w95:errorcluster, "item node ID"=w94:T2, "OPC UA server refnum out"=w93:T5)  [unwired: 3 in, 1 out]
          n93 = for {
            tunnel: w95 -> [w114]
            tunnel: w94 -> [w113]
            tunnel: w93 -> [w112]
            tunnel: [w111] -> w92 mode=indexing
            tunnel: w91 -> [w110] mode=indexing
            tunnel: [w109] -> w90 mode=indexing
            n94 = call "OPC Set Properties Name.vi"("error in (no error)"=w114, "name"=w110, "item node ID"=w113, "Refnum in"=w112) -> ("error out"=w111:errorcluster, "OPC Property cluster"=w109:T72)  [unwired: 6 in]
          }
          n95 = call "OPC Set Properties Name.vi"("error in (no error)"=w95, "name"=w99, "item node ID"=w94, "Refnum in"=w93) -> ("error out"=w98:errorcluster, "OPC Property cluster"=w97:T72)  [unwired: 6 in]
          n96 = Build Array (concatenate)(w97, w90) -> (w96:T4)
          n97 = Merge Errors(w98, w92) -> (w100:errorcluster)
        }
        n98 = Merge Errors(w39, w50) -> (w49:errorcluster)
        n99 = Merge Errors(w39, w48) -> (w47:errorcluster)
        n100 = Merge Errors(w39, w40) -> (w38:errorcluster)
        n101 = Merge Errors(w39, w52) -> (w51:errorcluster)
        n102 = Merge Errors(w39, w54) -> (w53:errorcluster)
        n103 = Merge Errors(w39, w46) -> (w45:errorcluster)
        n104 = Merge Errors(w39, w42) -> (w41:errorcluster)
        n105 = Merge Errors(w39, w44) -> (w43:errorcluster)
        n106 = Merge Errors(w38, w41, w43, w45, w47, w49, w51, w53) -> (w75:errorcluster)
        n107 = call <vilib>:"Start.vi"("error in (no error)"=w75, "OPC UA server refnum in"=w57) -> ("error out"=w84:errorcluster, "OPC UA server refnum out"=w85:T5)  [unwired: 7 in, 1 out]
        n108 = Build Array (concatenate)(w69, w68, w67, w66, w65, w63, w62, w61) -> (w64:T4)
      }
      frame "Exit" {
        n109 = case shown="True" w291 {
          tunnel: w297 -> [w300 w306]
          tunnel: [w300 w305] -> w296
          tunnel: w295 -> [w301 w304]
          tunnel: [w301 w303] -> w294
          tunnel: w293 -> [w299 w302]
          tunnel: [w299 w302] -> w290
          frame False {
          }
          frame True {
            # "7."
            # "6."
            # "5."
            n110 = call <vilib>:"Stop.vi"("error in (no error)"=w306, "OPC UA server refnum in"=w304) -> ("error out"=w308:errorcluster, "OPC UA server refnum out"=w309:T5)  [unwired: 8 in]
            n111 = call <vilib>:"Delete Node.vi"("error in (no error)"=w308, "node ID"=w302, "OPC UA server refnum in"=w309) -> ("error out"=w310:errorcluster, "OPC UA server refnum out"=w303:T5)  [unwired: 7 in]
            n112 = call <vilib>:"Close.vi"("error in (no error)"=w310, "OPC UA server refnum in"=w303) -> ("error out"=w307:errorcluster)  [unwired: 9 in]
            n113 = call <vilib>:"Simple Error Handler.vi"("error in (no error)"=w307) -> ("error out"=w305:errorcluster)  [unwired: 4 in, 4 out]
          }
        }
      }
      frame "Log" {
        n114 = call "Tag FGV.vi"("Operation"=Tag_FGV_Operation_Enum."Read All Tags", "error in (no error)"=w321) -> ("Tag Names"=w323:string[], "Tag Values"=w314:dbl[], "error out"=w320:errorcluster)  [unwired: 6 in, 5 out]
        "Tag Values" <- w314
        "Tag Names" <- w323
        n115 = for {
          tunnel: w323 -> [w335]
          tunnel: w320 -> [w330]
          tunnel: w319 -> [w336] mode=indexing
          tunnel: [w336] -> w318 mode=indexing
          tunnel: w317 -> [w331]
          tunnel: [w329] -> w316 mode=indexing
          tunnel: w314 -> [w328]
          tunnel: [w326] -> w313 mode=indexing
          tunnel: [w325] -> w312
          n116 = Unbundle By Name(w336) -> ("name"=w334:string, "property node ID"=w332:T2)
          n117 = Search 1D Array(1D array=w335, element=w334) -> (index of element=w333:i32)  [unwired: 1 in]
          n118 = Index Array(array=w328, index=w333) -> (element=w327:dbl)
          n119 = call-poly <vilib>:"Write.vi"("error in (no error)"=w330, "value"=w327, "node ID"=w332, "OPC UA server refnum in"=w331) -> ("error out"=w329:errorcluster, "status"=w326:T6, "OPC UA server refnum out"=w325:T5)  [unwired: 5 in]
        }
        "Array" <- w318
        "Array 2" <- w313
        n120 = Merge Errors(w316) -> (w315:errorcluster)
        "OPC UA server refnum out" <- w317
      }
    }
    "OPC UA server refnum out 3" <- w24
    "Array 3" <- w19
  }
